vi "Window-ROI group visualisation.vi"(8 "error in (no error)":errorcluster) -> (0 "error out":errorcluster)   [LabVIEW 2017]
uses:
  <vilib>/Utility/miscctls.llb/LVPointTypeDef.ctl
  User Interface/Visualisation/Functional Imaging Viewer/SubVIs/ROI grouping window/Globals/gl_ROI grp window globals.vi
  Global Variables/General Globals.vi
  User Interface/Visualisation/Functional Imaging Viewer/Global variables/gl_Functional Imaging-Global variables.vi
panel:
  out "Image":T1(plugin-control)
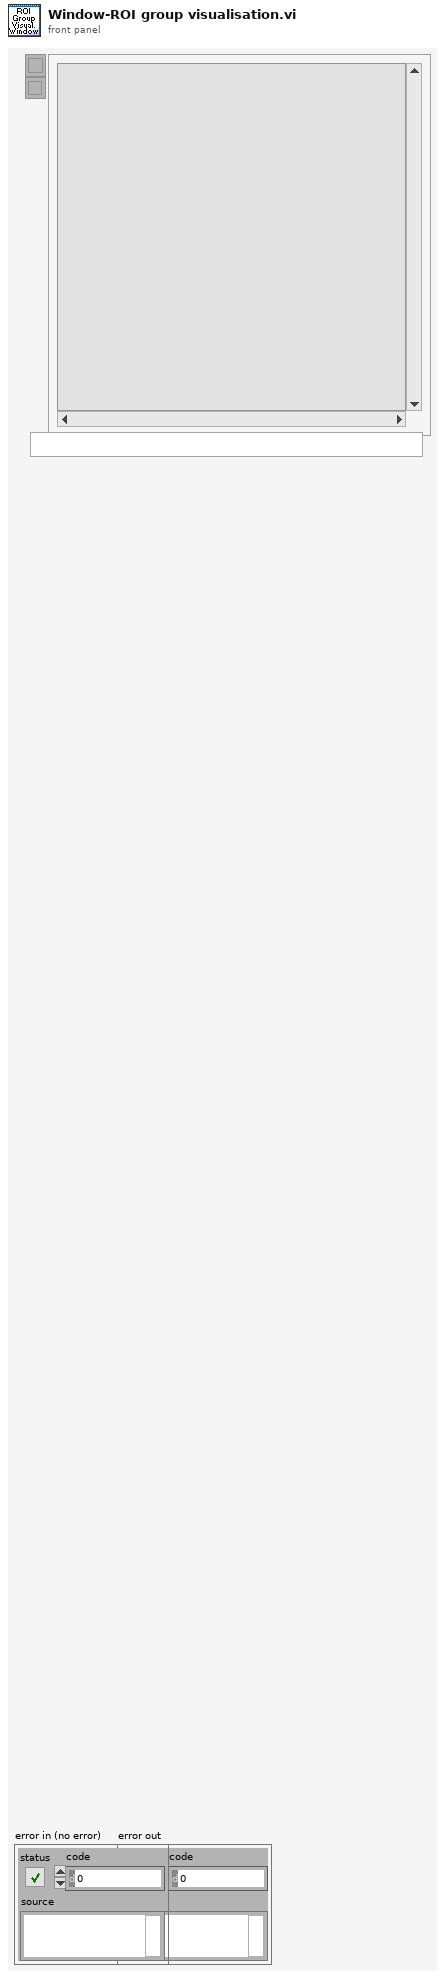
[diagram p1: front panel]
types:
  T1 = typedef "IMAQ Image.ctl" = refnum<image>
  T2 = typedef "LVPointTypeDef.ctl" = cluster{"Horizontal":i16, "Vertical":i16}
  T3 = typedef "ROI group info cluster.ctl" = cluster{"Group name":string, "# ROI in group":i32, "ROI numbers in group":i32[], "Group region specifier cluster":T4}
  T4 = typedef "ROI Descriptor" = cluster{"Global Rectangle":i32[], "Contours":cluster{"ID":enum32{"External", "Internal"}, "Type":u32, "Coordinates":i32[]}[]}
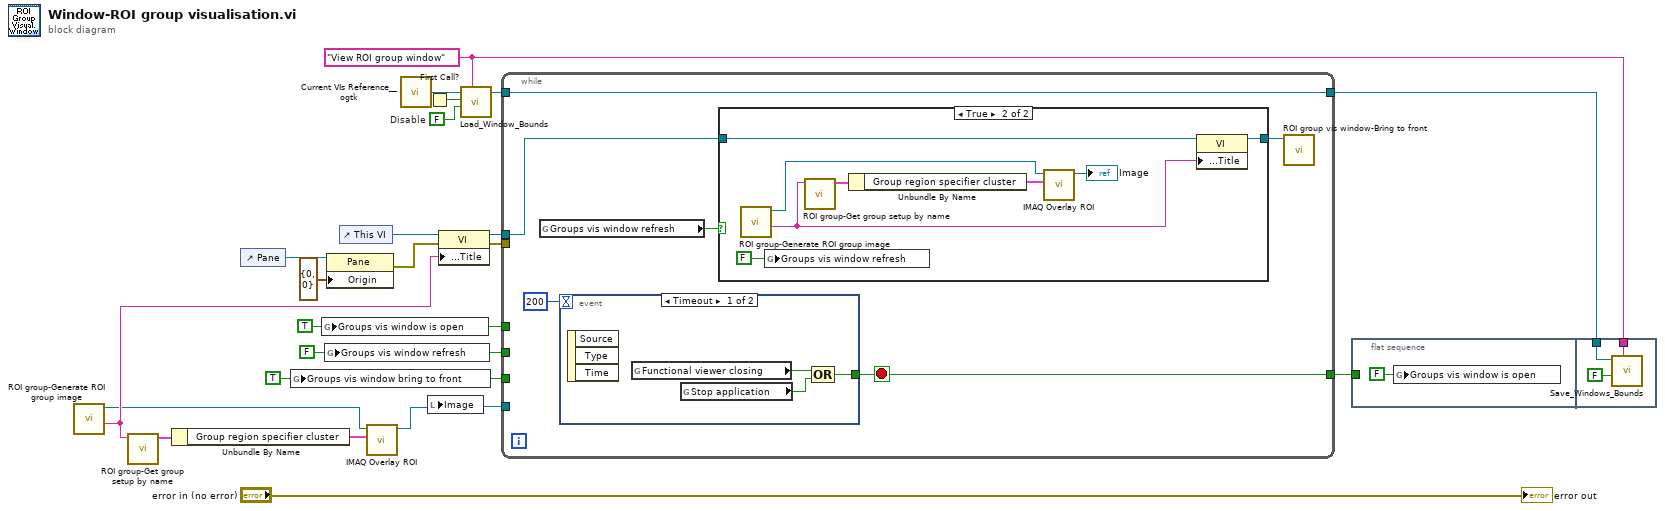
[diagram p0: block diagram]
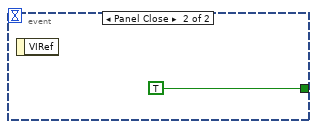
[diagram p3: hidden frame]
diagram:
  w6 = TRUE ("Bring to front")
  w8 = FALSE ("Groups vis window refresh")
  w10 = TRUE ("Groups vis window is open")
  w15 = FALSE  # Disable
  w11 = "View ROI group window" ("Window Name (i.e. Key)")
  n1 = call "ROI group-Generate ROI group image.vi"() -> ("Group Name"=w2:string, "Image to display"=w1:T1)  [unwired: 8 in, 2 out]
  n2 = call "ROI group-Get group setup by name.vi"("Name of ROI group to search for"=w2) -> ("POI group info cluster"=w5:T3)  [unwired: 8 in, 2 out]
  n3 = Unbundle By Name(w5) -> ("Group region specifier cluster"=w4:T4)
  n4 = control-ref of="Pane"() -> (w21:refnum<vi>)
  n5 = global write "gl_ROI grp window globals.vi" "Groups vis window bring to front"(w6) -> ()
  n6 = global write "gl_ROI grp window globals.vi" "Groups vis window is open"(w10) -> ()
  n7 = global write "gl_ROI grp window globals.vi" "Groups vis window refresh"(w8) -> ()
  n8 = property on="Property Node" class="Pane"(reference=w21, "Origin"=T2 {"Horizontal"=0, "Vertical"=0}) -> (error out=w19:errorcluster)  [unwired: 1 in, 1 out]
  n9 = control-ref of="This VI"() -> (w20:refnum<vi>)
  n10 = call "IMAQ Overlay ROI"("ROI Descriptor"=w4, "Image"=w1) -> ("Image Out"=w3:T1)  [unwired: 8 in, 1 out]
  n11 = call <userlib>:"Current VIs Reference__ogtk.vi"() -> ("Current VI's reference"=w17:refnum<vi>)  [unwired: 5 in]
  n12 = First Call?() -> (First Call?: T/F=w16:bool)
  n13 = local write "Image"(w3) -> ()
  n14 = property on="Property Node" class="VI"(reference=w20, error in=w19, "Front Panel.Title"=w2) -> (reference out=w7:refnum<vi>, error out=w18:errorcluster)
  n15 = call "Load_Window_Bounds.vi"("Window Name (i.e. Key)"=w11, "Disable"=w15, "First Call"=w16, "Window VI's Ref"=w17) -> ("reference out"=w14:refnum<vi>)  [unwired: 4 in, 3 out]
  n16 = while {
    tunnel: w3 -> [_]
    tunnel: w18 -> [_]
    tunnel: w14 -> [w27]
    tunnel: [w27] -> w12
    tunnel: [w26] -> w13
    tunnel: w10 -> [_]
    tunnel: w8 -> [_]
    tunnel: w7 -> [w24]
    tunnel: w6 -> [_]
    stop <- w26 stop-if-true
    n17 = global read "gl_ROI grp window globals.vi" "Groups vis window refresh"() -> (w25:bool)
    n18 = event shown="[0] Timeout" {
      selector: _ -> [_ _]
      dyn-events: _ -> [_ _]
      timeout: 200 -> [_ _]
      tunnel: [w38 TRUE ("Close")] -> w26
      event Timeout {
        n19 = event-data() -> ()  [unwired: 1 in, 3 out]
        n20 = global read "gl_Functional Imaging-Global variables.vi" "Functional viewer closing"() -> (w40:bool)
        n21 = global read "General Globals.vi" "Stop application"() -> (w39:bool)
        n22 = Compound Arithmetic op=OR(w40, w39) -> (w38:bool)
      }
      event Panel Close {
        n23 = event-data() -> ()  [unwired: 1 in, 1 out]
      }
    }
    n24 = case shown="True" w25 {
      tunnel: w24 -> [w29 w36]
      tunnel: [w29 w35] -> w23
      frame False {
      }
      frame True {
        n25 = call "ROI group-Generate ROI group image.vi"() -> ("Group Name"=w30:string, "Image to display"=w32:T1)  [unwired: 8 in, 2 out]
        n26 = global write "gl_ROI grp window globals.vi" "Groups vis window refresh"(FALSE ("Groups vis window refresh")) -> ()
        n27 = call "ROI group-Get group setup by name.vi"("Name of ROI group to search for"=w30) -> ("POI group info cluster"=w34:T3)  [unwired: 8 in, 2 out]
        n28 = Unbundle By Name(w34) -> ("Group region specifier cluster"=w33:T4)
        n29 = call "IMAQ Overlay ROI"("ROI Descriptor"=w33, "Image"=w32) -> ("Image Out"=→"Image":T1)  [unwired: 8 in, 1 out]
        n30 = property on="Property Node" class="VI"(reference=w36, "Front Panel.Title"=w30) -> (reference out=w35:refnum<vi>)  [unwired: 1 in, 1 out]
      }
    }
    n31 = call "ROI group vis window-Bring to front.vi"("VI's reference"=w23) -> ()  [unwired: 11 in]
  }
  n32 = flat-sequence {
    tunnel: w13 -> [_]
    tunnel: w12 -> [w44]
    tunnel: w11 -> [w43]
    frame #0 {
      n33 = global write "gl_ROI grp window globals.vi" "Groups vis window is open"(FALSE ("Groups vis window is open")) -> ()
    }
    frame #1 {
      n34 = call "Save_Windows_Bounds.vi"("Window Name (i.e. Key)"=w43, "Front Panel Window:Open"=FALSE, "Window VI's Ref"=w44) -> ()  [unwired: 8 in, 1 out]
    }
  }
  "error out" <- "error in (no error)"
